vi "Interpret Joysticks.vi"(10 "Joystick Controls":T4={"Driver Left Joystick X"=0.0, "Driver Left Joystick Y"=0.0, "Driver A Button"=FALSE, "Driver B Button"=FALSE, "Driver X Button"=FALSE, "Driver Y Button"=FALSE, "Driver Left Bumper"=FALSE, "Driver Right Bumper"=FALSE, "Driver View Button"=FALSE, "Driver Menu Button"=FALSE, "Driver Left Joystick Press"=FALSE, "Driver Right Joystick Press"=FALSE, "Driver Left Trigger"=0.0, "Driver Right Joystick X"=0.0, "Driver Right Joystick Y"=0.0, "Driver Right Trigger"=0.0, "Operator Left Joystick X"=0.0, "Operator Left Joystick Y"=0.0, "Operator A Button"=FALSE, "Operator B Button"=FALSE, "Operator X Button"=FALSE, "Operator Y Button"=FALSE, "Operator Left Bumper"=FALSE, "Operator Right Bumper"=FALSE, "Operator View Button"=FALSE, "Operator Menu Button"=FALSE, "Operator Left Joystick Press"=FALSE, "Operator Right Joystick Press"=FALSE, "Operator Left Trigger"=0.0, "Operator Right Joystick X"=0.0, "Operator Right Joystick Y"=0.0, "Operator Right Trigger"=0.0, "Driver D-Pad"=-1, "Operator D-Pad"=-1}) -> (1 "Teleop Hatch and Cargo":T1, 2 "4bar output":T3 {"Control Mode" items=["PercentOutput"=0, "Position"=1, "Velocity"=2, "Current"=3, "Follower"=5, "MotionProfile"=6, "MotionMagic"=7, "MotionProfileArc"=10, "Disabled"=15]}, 3 "Drive Motor Values":cluster{"Left Motor":dbl, "Right Motor":dbl})   [LabVIEW 2018]
uses:
  Joystick Controls.ctl
  <vilib>/Rock Robotics/WPI/ThirdParty/Phoenix-LabVIEW/Motor Controller/Controls/CTRE_Phoenix_MotorControl_ControlMode.ctl
  Robot Global Data.vi
panel:
  # "NOT DONE"
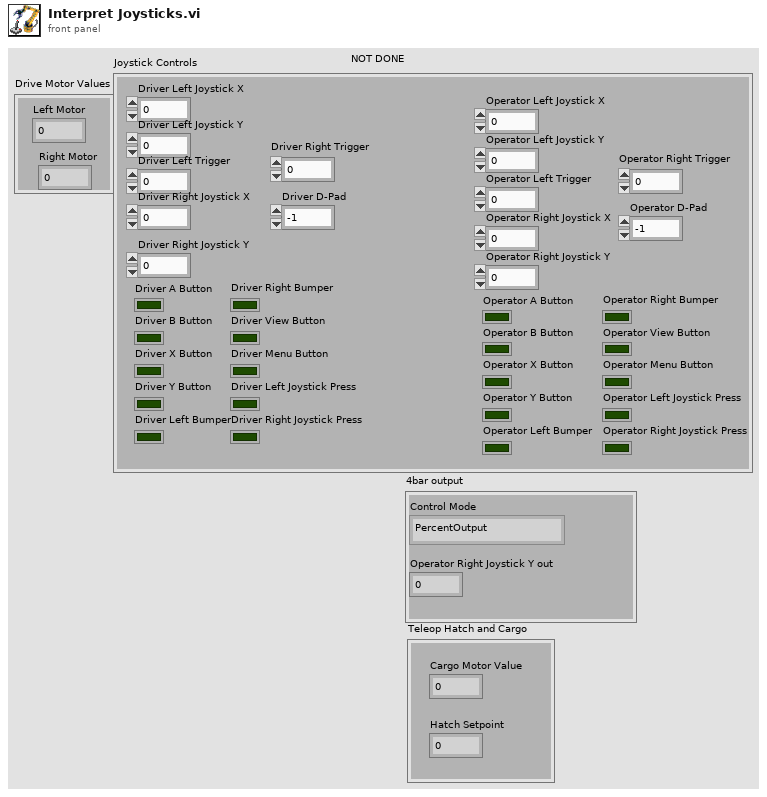
[diagram p1: front panel]
types:
  T1 = cluster{"Cargo Motor Value":dbl, "Hatch Setpoint":dbl}
  T2 = typedef "CTRE_Phoenix_MotorControl_ControlMode.ctl" = u16
  T3 = cluster{"Control Mode":T2, "Operator Right Joystick Y out":dbl}
  T4 = typedef "Joystick Controls.ctl" = cluster{"Driver Left Joystick X":dbl, "Driver Left Joystick Y":dbl, "Driver A Button":bool, "Driver B Button":bool, "Driver X Button":bool, "Driver Y Button":bool, "Driver Left Bumper":bool, "Driver Right Bumper":bool, "Driver View Button":bool, "Driver Menu Button":bool, "Driver Left Joystick Press":bool, "Driver Right Joystick Press":bool, "Driver Left Trigger":dbl, "Driver Right Joystick X":dbl, "Driver Right Joystick Y":dbl, "Driver Right Trigger":dbl, "Operator Left Joystick X":dbl, "Operator Left Joystick Y":dbl, "Operator A Button":bool, "Operator B Button":bool, "Operator X Button":bool, "Operator Y Button":bool, "Operator Left Bumper":bool, "Operator Right Bumper":bool, "Operator View Button":bool, "Operator Menu Button":bool, "Operator Left Joystick Press":bool, "Operator Right Joystick Press":bool, "Operator Left Trigger":dbl, "Operator Right Joystick X":dbl, "Operator Right Joystick Y":dbl, "Operator Right Trigger":dbl, "Driver D-Pad":i16, "Operator D-Pad":i16}
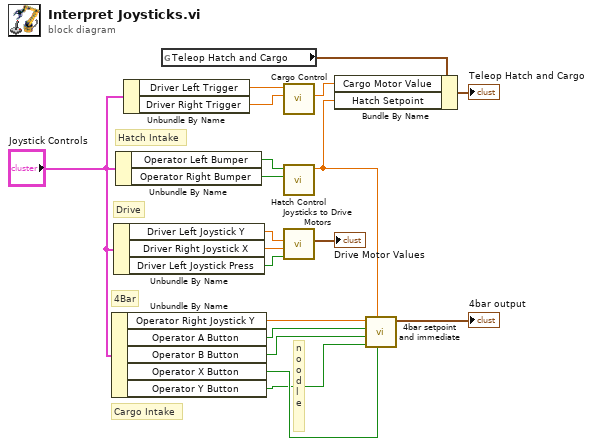
[diagram p0: block diagram]
diagram:
  # "n\no\no\nd\nl\ne"
  # "Hatch Intake"
  # "Cargo Intake"
  # "4Bar"
  # "Drive"
  n1 = Unbundle By Name("Joystick Controls") -> ("Operator Right Joystick Y"=w14:dbl, "Operator A Button"=w13:bool, "Operator B Button"=w12:bool, "Operator X Button"=w11:bool, "Operator Y Button"=w10:bool)
  n2 = Unbundle By Name("Joystick Controls") -> ("Driver Left Joystick Y"=w16:dbl, "Driver Right Joystick X"=w17:dbl, "Driver Left Joystick Press"=w18:bool)
  n3 = Unbundle By Name("Joystick Controls") -> ("Operator Left Bumper"=w3:bool, "Operator Right Bumper"=w2:bool)
  n4 = Unbundle By Name("Joystick Controls") -> ("Driver Left Trigger"=w8:dbl, "Driver Right Trigger"=w7:dbl)
  n5 = global read "Robot Global Data.vi" "Teleop Hatch and Cargo"() -> (w5:T1)
  n6 = call "Cargo Control.vi"("Operator Right Trigger"=w7, "Operator Left Trigger"=w8) -> ("Numeric"=w6:dbl)  [unwired: 9 in]
  n7 = call "Hatch Control.vi"("Driver Right Bumper"=w2, "Driver Left Bumper"=w3) -> ("Hatch Intake Floor"=w1:dbl)  [unwired: 9 in]
  n8 = call "Joysticks to Drive Motors.vi"("Boost?"=w18, "Turn"=w17, "Throttle"=w16) -> ("Drive Motor Values"=→"Drive Motor Values":cluster{"Left Motor":dbl, "Right Motor":dbl})  [unwired: 8 in]
  n9 = Bundle By Name(cluster=w5, "Cargo Motor Value"=w6, "Hatch Setpoint"=w1) -> (→"Teleop Hatch and Cargo":T1)
  n10 = call "4bar setpoint and immediate.vi"("Operator X Button"=w11, "Hatch Setpoint"=w1, "Operator Y Button"=w10, "Operator B Button"=w12, "Operator A Button"=w13, "Operator Right Joystick Y in"=w14) -> ("Output"=→"4bar output":T3)  [unwired: 5 in]
